vi "panel_update_status_string.vi"(8 "error in (no error)":errorcluster, 10 "String":string, 11 "scan_panel in":refnum<class "scan_panel.lvclass">) -> (0 "error out":errorcluster, 3 "scan_panel out":refnum<class "scan_panel.lvclass">)   [LabVIEW 2015, in "scan_panel.lvclass"]
uses:
  scan_panel.lvclass
  scan_panel.lvclass/scan_panel.ctl
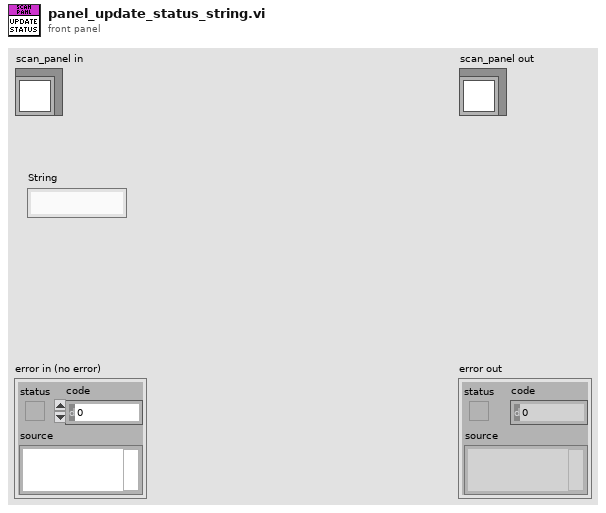
[diagram p1: front panel]
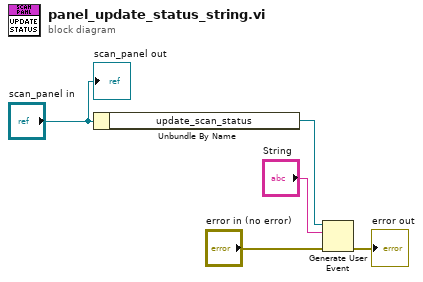
[diagram p0: block diagram]
diagram:
  n1 = Unbundle By Name("scan_panel in") -> ("update_scan_status"=w5:refnum<user-event>)
  n2 = Generate User Event(user event=w5, event data cluster="String", error in="error in (no error)") -> (error out=→"error out":errorcluster)  [unwired: 1 in, 1 out]
  "scan_panel out" <- "scan_panel in"
